vi "Read Movement Ratios.vi"(2 "error in (no error)":errorcluster, 3 "Car.lvclass":refnum<class "Car.lvclass">) -> (0 "error out":errorcluster, 1 "Array":dbl[](array[numeric]))   [LabVIEW 2015, in "Car.lvclass"]
uses:
  Car.lvclass
  Car.lvclass/Car.ctl
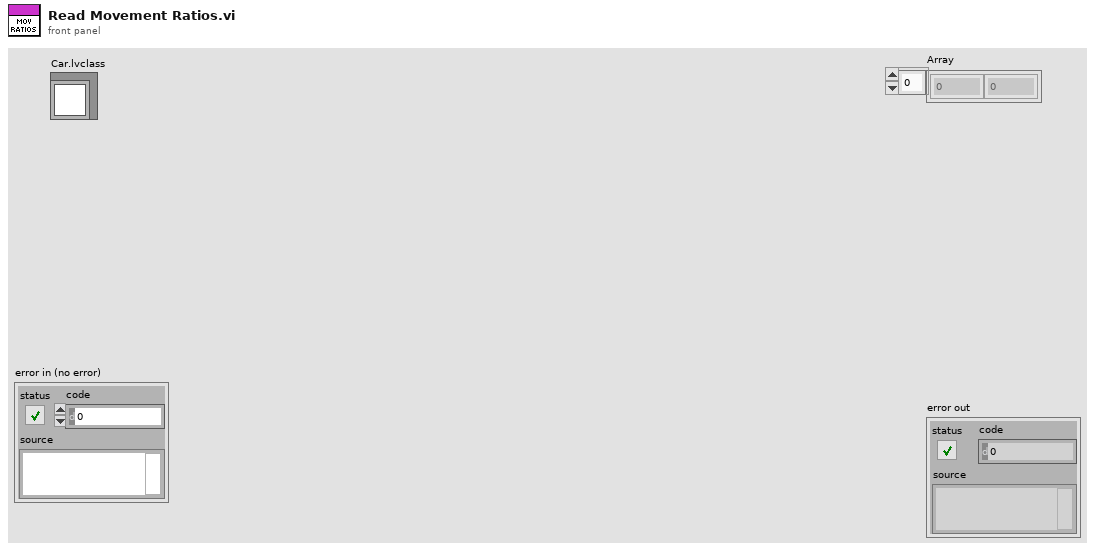
[diagram p1: front panel]
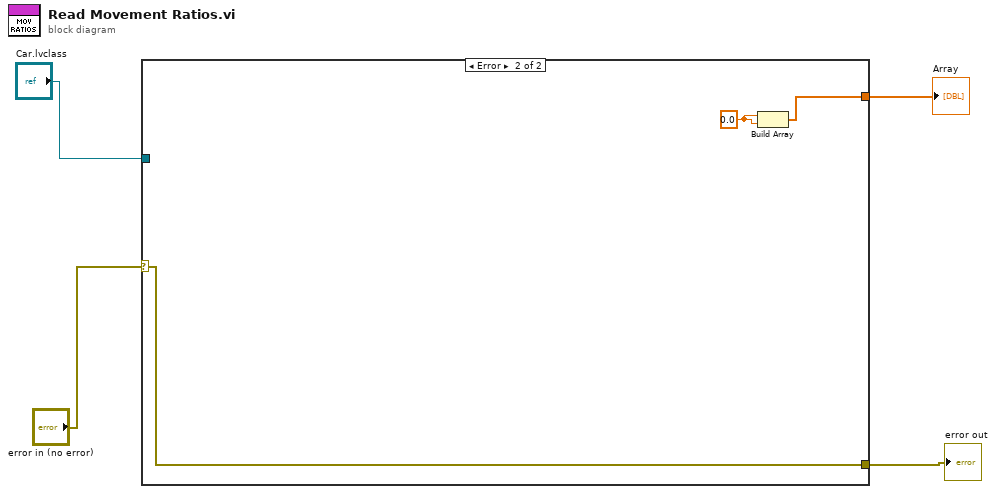
[diagram p0: block diagram]
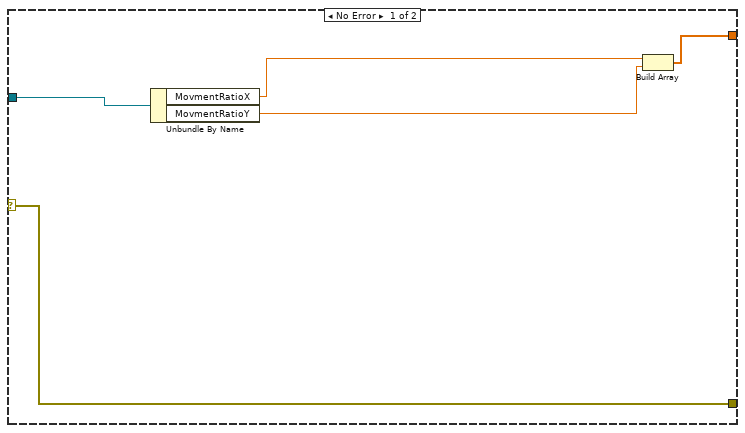
[diagram p2: hidden frame]
diagram:
  n1 = case shown="Error" "error in (no error)" {
    selector: "error in (no error)" -> [w9 w12]
    tunnel: [w9 w12] -> w3
    tunnel: "Car.lvclass" -> [w8 _]
    tunnel: [w5 w11] -> w1
    frame No Error {
      n2 = Unbundle By Name(w8) -> ("MovmentRatioX"=w7:dbl, "MovmentRatioY"=w6:dbl)
      n3 = Build Array(w7, w6) -> (w5:dbl[])
    }
    frame Error {
      w10 = 0.0
      n4 = Build Array(w10, w10) -> (w11:dbl[])
    }
  }
  "error out" <- w3
  "Array" <- w1
